vi "GetCompiledSettingsDialog.vi"(11 "Cluster":T1 {"IncomingRegisters.Settings"."Register"."Data Type" format="%.0x"; "IncomingRegisters.Refs"."Refs"."Data Reference" format="%.0x"; "OutgoingRegisters.Settings"."Register"."Data Type" format="%.0x"; "OutgoingRegisters.Refs"."Refs"."Data Reference" format="%.0x"; "IncomingDMA.Settings"."DMA.Settings"."dt" format="%#_p"; "IncomingDMA.Settings"."DMA.Settings"."Update Rate" items=["1 Hz"=1, "2 Hz"=2, "5 Hz"=5, "10 Hz"=10]; "IncomingDMA.Settings"."WritetoVSEngine.Refs"."Refs" format="%.0x"; "OutgoingDMA.Settings"."DMA.Settings"."dt" format="%#_p"; "OutgoingDMA.Settings"."DMA.Settings"."Update Rate" items=["1 Hz"=1, "2 Hz"=2, "5 Hz"=5, "10 Hz"=10]; "OutgoingDMA.Settings"."WritetoVSEngine.Refs"."Refs" format="%.0x"}) -> (3 "output cluster":T1 {"IncomingRegisters.Settings"."Register"."Data Type" format="%.0x"; "IncomingRegisters.Refs"."Refs"."Data Reference" format="%.0x"; "OutgoingRegisters.Settings"."Register"."Data Type" format="%.0x"; "OutgoingRegisters.Refs"."Refs"."Data Reference" format="%.0x"; "IncomingDMA.Settings"."DMA.Settings"."dt" format="%#_p"; "IncomingDMA.Settings"."DMA.Settings"."Update Rate" items=["1 Hz"=1, "2 Hz"=2, "5 Hz"=5, "10 Hz"=10]; "IncomingDMA.Settings"."WritetoVSEngine.Refs"."Refs" format="%.0x"; "OutgoingDMA.Settings"."DMA.Settings"."dt" format="%#_p"; "OutgoingDMA.Settings"."DMA.Settings"."Update Rate" items=["1 Hz"=1, "2 Hz"=2, "5 Hz"=5, "10 Hz"=10]; "OutgoingDMA.Settings"."WritetoVSEngine.Refs"."Refs" format="%.0x"})   [LabVIEW 2013, in "FPGA Addon System Explorer.lvlib"]
uses:
  FPGA Addon System Explorer.lvlib
  Shared/Compiled.Settings
  Shared/Compiled.RegisterSettings.ctl
  Shared/Scalar Type.ctl
  Shared/Register Information.ctl
  <userlib>/_OpenG.lib/lvdata/lvdata.llb/Type Descriptor Enumeration__ogtk.ctl
  <vilib>/NI Veristand/Custom Device API/Block Data Reference.ctl
  <vilib>/NI Veristand/Custom Device API/Data Reference.ctl
  Shared/Compiled.DMASettings.ctl
  Shared/DMA Settings.ctl
  Shared/Delacing Scheme.ctl
  <vilib>/NI Veristand/Custom Device API/Waveform Data Reference.ctl
  Shared/FPGA Settings.ctl
  <vilib>/NI VeriStand/Custom Device API/Custom Device API.lvlib
  Shared/FPGA Addon Shared.lvlib
panel:
  in  "OK Button":bool
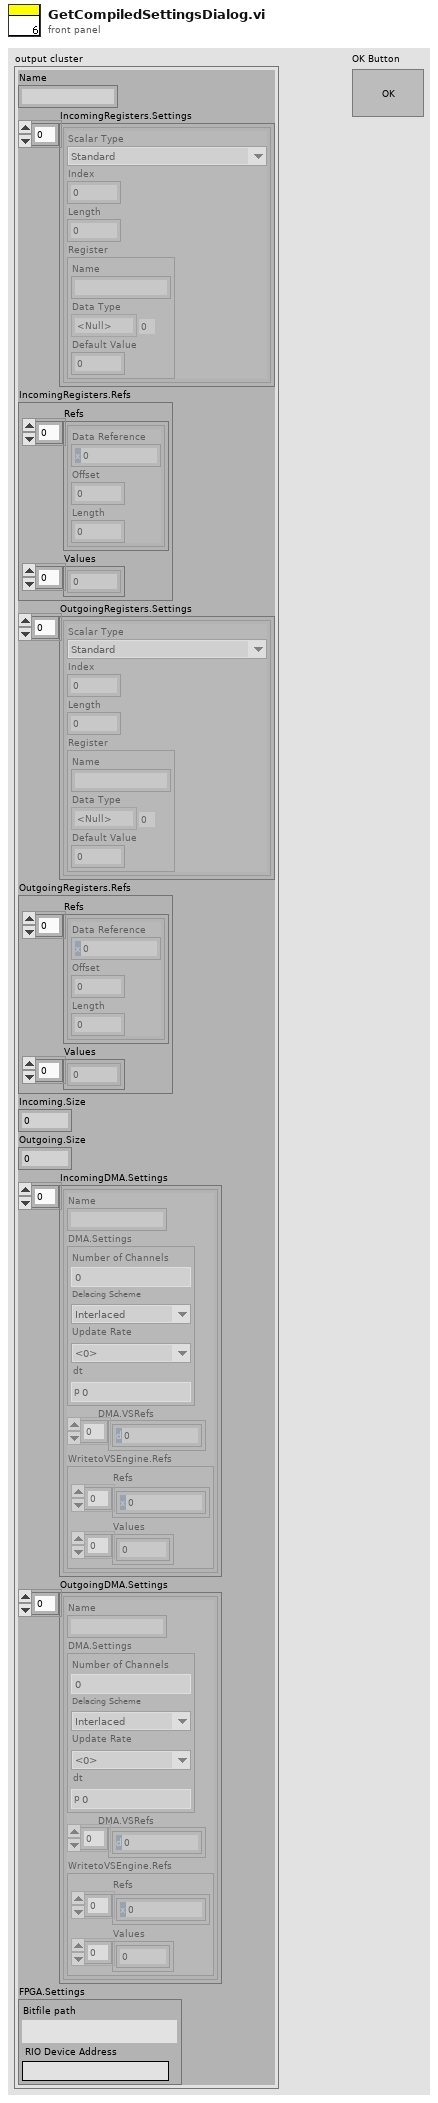
[diagram p1: front panel]
types:
  T1 = typedef "FPGA Addon Shared.lvlib/Compiled.Settings" = cluster{"Name":string, "IncomingRegisters.Settings":T2[], "IncomingRegisters.Refs":cluster{"Refs":T6[], "Values":dbl[]}, "OutgoingRegisters.Settings":T2[], "OutgoingRegisters.Refs":cluster{"Refs":T6[], "Values":dbl[]}, "Incoming.Size":i32, "Outgoing.Size":i32, "IncomingDMA.Settings":T8[], "OutgoingDMA.Settings":T8[], "FPGA.Settings":T12}
  T2 = typedef "FPGA Addon Shared.lvlib/Compiled.RegisterSettings.ctl" = cluster{"Scalar Type":T3, "Index":i32, "Length":i32, "Register":T4}
  T3 = typedef "FPGA Addon Shared.lvlib/Scalar Type.ctl" = enum16{"Standard", "Bitpacked"}
  T4 = typedef "FPGA Addon Shared.lvlib/Register Information.ctl" = cluster{"Name":string, "Data Type":T5, "Default Value":dbl}
  T5 = typedef "Type Descriptor Enumeration__ogtk.ctl" = enum8{"<Null>", "I8", "I16", "I32", "I64", "U8", "U16", "U32", "U64", "SGL", "DBL", "EXT", "CSG", "CDB", "CXT", "0x0F", "0x10", "0x11", "0x12", "0x13", "0x14", "Enum U8", "Enum U16", "Enum U32", "Enum U64", "SGL PQ", "DBL PQ", "EXT PQ", "CSG PQ", "CDB PQ", "CXT PQ", "0x1F", "0x20", "Boolean", "0x22", "0x23", "0x24", "0x25", "0x26", "0x27", "0x28", "0x29", "0x2A", "0x2B", "0x2C", "0x2D", "0x2E", "0x2F", "String", "0x31", "Path", "Pict", "0x34", "0x35", "0x36", "DAQ", "0x38", "0x39", "0x3A", "0x3B", "0x3C", "0x3D", "0x3E", "0x3F", "Array", "0x41", "0x42", "0x43", "0x44", "0x45", "0x46", "0x47", "0x48", "0x49", "0x4A", "0x4B", "0x4C", "0x4D", "0x4E", "0x4F", "Cluster", "0x51", "0x52", "Variant", "Waveform", "0x55", "0x56", "0x57", "0x58", "0x59", "0x5A", "0x5B", "0x5C", "0x5D", "0x5E", "0x5F", "0x60", "0x61", "0x62", "0x63", "0x64", "0x65", "0x66", "0x67", "0x68", "0x69", "0x6A", "0x6B", "0x6C", "0x6D", "0x6E", "0x6F", "Refnum"}
  T6 = typedef "Custom Device API.lvlib/Block Data Reference.ctl" = cluster{"Data Reference":T7, "Offset":i32, "Length":i32}
  T7 = typedef "Custom Device API.lvlib/Data Reference.ctl" = i32
  T8 = typedef "FPGA Addon Shared.lvlib/Compiled.DMASettings.ctl" = cluster{"Name":string, "DMA.Settings":T9, "DMA.VSRefs":T11[], "WritetoVSEngine.Refs":cluster{"Refs":T7[], "Values":dbl[]}}
  T9 = typedef "FPGA Addon Shared.lvlib/DMA Settings.ctl" = cluster{"Number of Channels":u8, "Delacing Scheme":T10, "Update Rate":u32, "dt":dbl}
  T10 = typedef "FPGA Addon Shared.lvlib/Delacing Scheme.ctl" = enum8{"Interlaced"}
  T11 = typedef "Custom Device API.lvlib/Waveform Data Reference.ctl" = i32
  T12 = typedef "FPGA Addon Shared.lvlib/FPGA Settings.ctl" = cluster{"Bitfile path":path, "RIO Device Address":string}
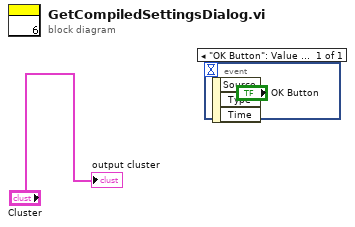
[diagram p0: block diagram]
diagram:
  n1 = event shown="[0] \"OK Button\": Value Change" {
    selector: _ -> [_]
    dyn-events: _ -> [_]
    timeout: _ -> [_]
    event "OK Button": Value Change {
      n2 = event-data() -> ()  [unwired: 1 in, 3 out]
    }
  }
  "output cluster" <- "Cluster"
